vi "Sort 2D Array (U8)__ogtk.vi"(6 "Column/Row to Sort By":u32, 8 "Sort By in":enum16{"row", "column"}(ring), 9 "Order":enum16{"ascending", "descending"}(ring), 11 "Array in":u8[][](array[numeric])) -> (0 "Sort By out":enum16{"row", "column"}(ring), 1 "Index Out of Range?":bool, 2 "Sorted Pointers":i32[](array[numeric]), 3 "Sorted Array out":u8[][](array[numeric]))   [LabVIEW 2012]
doc: "This polymorphic VI sorts a 2D array of numerics or strings, regardless of the array size. You can specify whether to sort by column or row, which column or row to sort by, and whether to sort in ascending or descending order. You also can specify a secondary row or column to sort by."
panel:
  # "Sort 2D Array\n\nThis VI sorts by row or by column, a 2D array of any size in descending or ascending order based on a column or row whose index you specify.\n\nPlease visit http://www.OpenG.org to learn about the\nOpen Source LabVIEW software movement.\n\nNOTICE -- YOU MUST LEAVE THIS NOTICE IN PLACE.  PER THE TERMS OF THE LICENSE BELOW, YOU MAY SUBLICENSE THIS SOFTWARE \nIN ANY WAY THAT DOES NOT CONFLICT WITH THIS LICENSE.\n\n### BSD License (http://www.opensource.org/licenses/bsd-license.php) Begin ###\n \nCopyright (c) 2002, Jim Kring <jim@jimkring.com>\nCopyright (c) 2002, Cal-Bay Systems, Inc. <info@calbay.com>\n\nAll rights reserved.\n\nRedistribution and use in source and binary forms, with or without modification, are permitted provided that the following conditions are met:\n\n    * Redistributions of source code must retain the above copyright notice, this list of conditions and the following disclaimer.\n    * Redistributions in binary form must reproduce the above copyright notice, this list of conditions and the following disclaimer in the \n       documentation and/or other materials provided with the distribution.\n    * Neither the name of SciWare, James Kring, Inc., nor the names of its contributors may be used to endorse or promote products derived \n       from this software without specific prior written permission.\n\nTHIS SOFTWARE IS PROVIDED BY THE COPYRIGHT HOLDERS AND CONTRIBUTORS \"AS IS\" AND ANY EXPRESS OR IMPLIED WARRANTIES, \nINCLUDING, BUT NOT LIMITED TO, THE IMPLIED WARRANTIES OF MERCHANTABILITY AND FITNESS FOR A PARTICULAR PURPOSE ARE \nDISCLAIMED. IN NO EVENT SHALL THE COPYRIGHT OWNER OR CONTRIBUTORS BE LIABLE FOR ANY DIRECT, INDIRECT, INCIDENTAL,\n SPECIAL, EXEMPLARY, OR CONSEQUENTIAL DAMAGES (INCLUDING, BUT NOT LIMITED TO, PROCUREMENT OF SUBSTITUTE GOODS OR \nSERVICES; LOSS OF USE, DATA, OR PROFITS; OR BUSINESS INTERRUPTION) HOWEVER CAUSED AND ON ANY THEORY OF LIABILITY, \nWHETHER IN CONTRACT, STRICT LIABILITY, OR TORT (INCLUDING NEGLIGENCE OR OTHERWISE) ARISING IN ANY WAY OUT OF THE USE \nOF THIS SOFTWARE, EVEN IF ADVISED OF THE POSSIBILITY OF SUCH DAMAGE.\n\n### BSD License End ###"
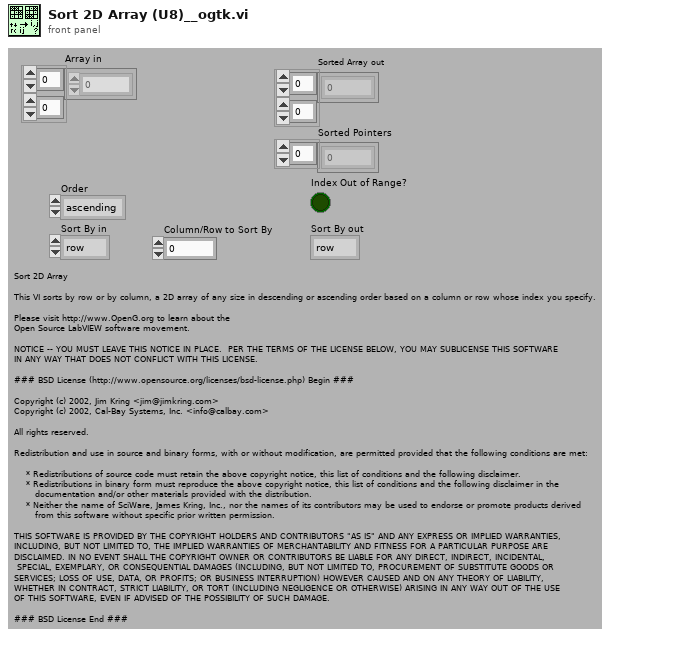
[diagram p1: front panel]
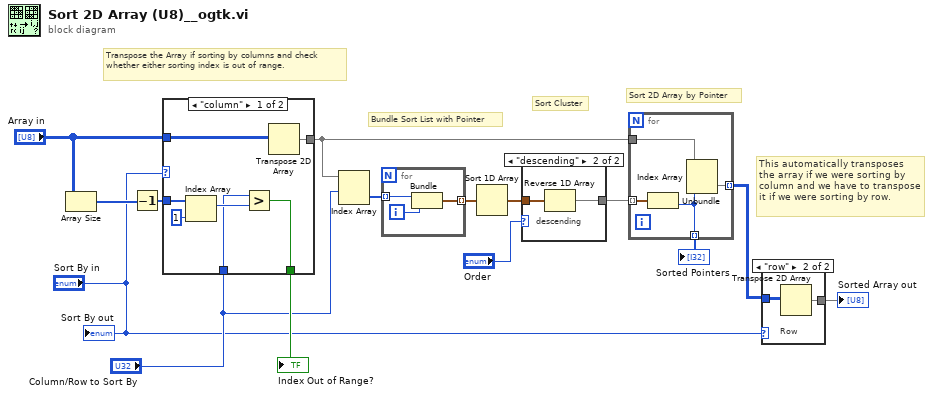
[diagram p0: block diagram]
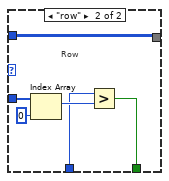
[diagram p4: hidden frame]
diagram:
  # "Sort 2D Array by Pointer"
  # "Sort Cluster"
  # "This automatically transposes the array if we were sorting by column and we have to transpose it if we were sorting by row."
  # "Bundle Sort List with Pointer"
  # "Transpose the Array if sorting by columns and check whether either sorting index is out of range."
  n1 = Array Size(array="Array in") -> (size(s)=w11:i32[])
  n2 = Decrement(x=w11) -> (x-1=w8:i32[])
  n3 = case shown="\"column\"" "Sort By in" {
    tunnel: "Array in" -> [w22 w28]
    tunnel: [w21 w28] -> w15
    tunnel: w8 -> [w20 w25]
    tunnel: [w16 w23] -> w10
    tunnel: "Column/Row to Sort By" -> [w17 w24]
    frame "column" {
      n4 = Index Array(array=w20, index=1 ("Index")) -> (element=w18:i32)
      n5 = Greater?(x=w17, y=w18) -> (0:w16:bool)
      n6 = Transpose 2D Array(2D array=w22) -> (transposed array=w21:u8[][])
    }
    frame "row" {
      # "Row"
      n7 = Index Array(array=w25, index=0 ("Index")) -> (element=w27:i32)
      n8 = Greater?(x=w24, y=w27) -> (0:w23:bool)
    }
  }
  "Index Out of Range?" <- w10
  n9 = Index Array(array=w15, index (row)="Column/Row to Sort By") -> (element=w5:u8[])  [unwired: 1 in]
  n10 = for {
    tunnel: w5 -> [w31] mode=indexing
    tunnel: [w29] -> w4 mode=indexing
    i -> [w30]
    n11 = Bundle("Numeric"=w31, w30) -> (w29:cluster{"Numeric":u8, i32})  [unwired: 1 in]
  }
  n12 = Sort 1D Array(array=w4) -> (sorted array=w3:cluster{"Numeric":u8, i32}[])
  n13 = case shown="\"descending\"" "Order" {
    tunnel: [w32 w33] -> w6
    tunnel: w3 -> [w32 w34]
    frame "ascending", Default {
    }
    frame "descending" {
      # "descending"
      n14 = Reverse 1D Array(array=w34) -> (reversed array=w33:cluster{"Numeric":u8, i32}[])
    }
  }
  n15 = for {
    tunnel: w6 -> [w38] mode=indexing
    tunnel: w15 -> [w37]
    tunnel: [w36] -> w14 mode=indexing
    tunnel: [w35] -> w2 mode=indexing
    n16 = Unbundle(w38) -> (w35:i32)  [unwired: 1 out]
    n17 = Index Array(array=w37, index (col)=w35) -> (element=w36:u8[])  [unwired: 1 in]
  }
  "Sorted Pointers" <- w2
  n18 = case shown="\"row\"" "Sort By in" {
    tunnel: w14 -> [w39 w41]
    tunnel: [w39 w40] -> w13
    frame "column" {
    }
    frame "row" {
      # "Row"
      n19 = Transpose 2D Array(2D array=w41) -> (transposed array=w40:u8[][])
    }
  }
  "Sorted Array out" <- w13
  "Sort By out" <- "Sort By in"
